vi "quack.vi"(8 "error in (no error)":errorcluster, 11 "Squeak in":refnum<class "Squeak.lvclass">) -> (0 "error out":errorcluster, 2 "String":string, 3 "Squeak out":refnum<class "Squeak.lvclass">)   [LabVIEW 2013, in "Squeak.lvclass"]
uses:
  Squeak.lvclass
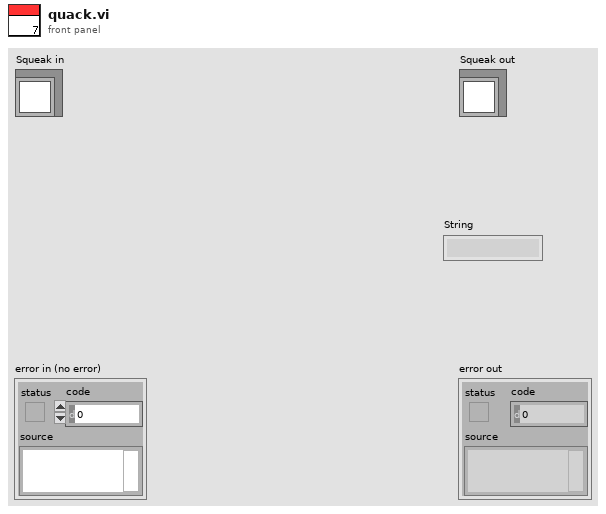
[diagram p1: front panel]
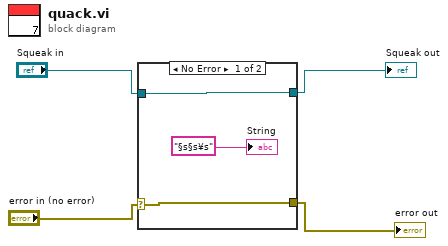
[diagram p0: block diagram]
diagram:
  n1 = case shown="No Error" "error in (no error)" {
    selector: "error in (no error)" -> [w7 w9]
    tunnel: [w7 w9] -> w2
    tunnel: [w6 w8] -> w3
    tunnel: "Squeak in" -> [w6 w8]
    frame No Error {
      "String" <- "§s§s¥s" ("String")
    }
    frame Error {
    }
  }
  "error out" <- w2
  "Squeak out" <- w3
